vi "dynResToPixelFormat.vi"(8 "error in (no error)":errorcluster, 10 "dyn_res":u32) -> (0 "error out":errorcluster, 2 "PixelFormat":u32)   [LabVIEW 2019, in "Camera.lvclass"]
doc: "Finds the pixel format for the specified dynamic resolution"
uses:
  Camera.lvclass
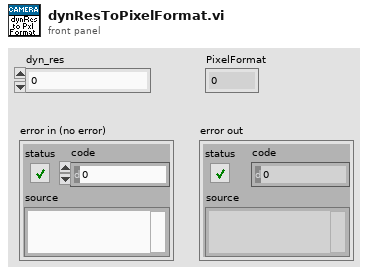
[diagram p1: front panel]
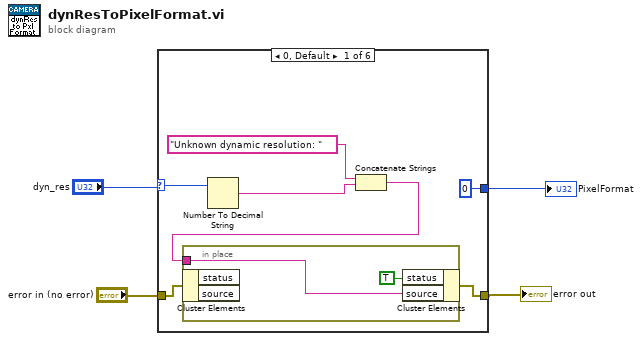
[diagram p0: block diagram]
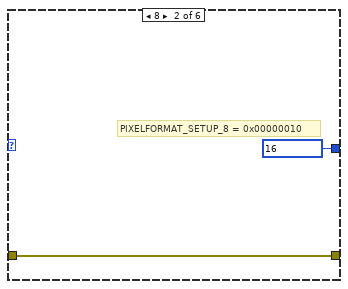
[diagram p2: hidden frame]
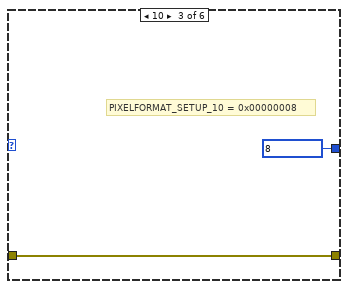
[diagram p3: hidden frame]
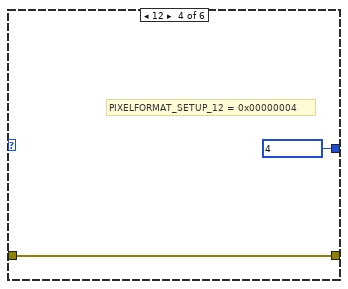
[diagram p4: hidden frame]
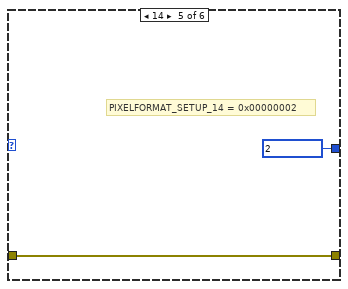
[diagram p5: hidden frame]
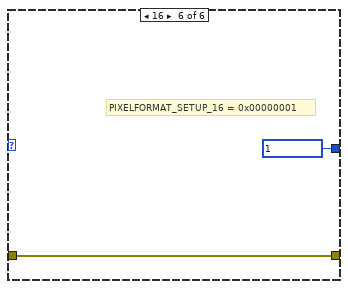
[diagram p6: hidden frame]
diagram:
  n1 = case shown="0, Default" "dyn_res" {
    selector: "dyn_res" -> [w8 _ _ _ _ _]
    tunnel: [u32 0 u32 16 u32 8 u32 4 u32 2 u32 1] -> w3
    tunnel: "error in (no error)" -> [w10 w14 w16 w18 w20 w22]
    tunnel: [w9 w14 w16 w18 w20 w22] -> w1
    frame 0, Default {
      n2 = Number To Decimal String(number=w8) -> (decimal integer string=w7:string)  [unwired: 1 in]
      n3 = Concatenate Strings("Unknown dynamic resolution: ", w7) -> (w5:string)
      n4 = in-place {
        in-place-border: w5 -> [w12]
        n5 = in-place-cluster #1(w10) -> ()  [unwired: 2 out]
        n6 = in-place-cluster #1("status"=TRUE, "source"=w12) -> (w9:errorcluster)
      }
    }
    frame 8 {
      # "PIXELFORMAT_SETUP_8 = 0x00000010"
    }
    frame 10 {
      # "PIXELFORMAT_SETUP_10 = 0x00000008"
    }
    frame 12 {
      # "PIXELFORMAT_SETUP_12 = 0x00000004"
    }
    frame 14 {
      # "PIXELFORMAT_SETUP_14 = 0x00000002"
    }
    frame 16 {
      # "PIXELFORMAT_SETUP_16 = 0x00000001"
    }
  }
  "PixelFormat" <- w3
  "error out" <- w1
